vi "XYZStage-Read speed setting command.vi"(8 "error in (no error)":errorcluster, 9 "XYZ Stage data to queue":T2={"Command"=enum."Initialize", "Channel"="Z", "X"=0.0, "Y"=0.0, "Z"=0.0, "Speed"=0, "Zero"=FALSE, "Use acknowledgement?"=TRUE} {"Speed" format="Speed= %.0f"; "Z" format="Z= %#_g"; "Y" format="Y= %#_g"; "X" format="X= %#_g"}, 10 "Z Stage":T1, 11 "XY Stage config cluster":T5) -> (0 "error out":errorcluster)   [LabVIEW 2020]
doc: "Reads the XYZ Stage coordinates"
uses:
  Typedefs/XY Stage config cluster.ctl
  Typedefs/XYZ stage data.ctl
  Typedefs/XYZ stage states.ctl
  Typedefs/XYZ channel ring.ctl
  Typedefs/Z Stage config cluster.ctl
  Typedefs/Command acknowledgment states.ctl
  Global Variables/General Globals.vi
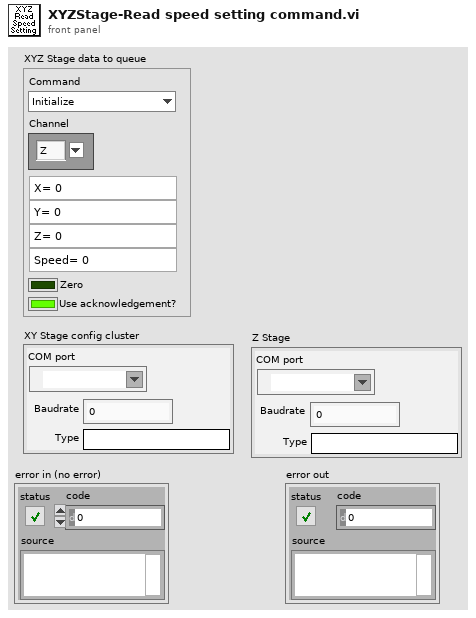
[diagram p1: front panel]
types:
  T1 = typedef "Z Stage config cluster.ctl" = cluster{"COM port":refnum<visa-resource-name>, "Baudrate":i32, "Type":string}
  T2 = typedef "XYZ stage data.ctl" = cluster{"Command":T3, "Channel":T4, "X":sgl, "Y":sgl, "Z":sgl, "Speed":i32, "Zero":bool, "Use acknowledgement?":bool}
  T3 = typedef "XYZ stage states.ctl" = enum16{"Dequeue", "Initialize", "Read Position", "Read Speed Setting", "Move", "Set Max Speed", "Reset Axis", "Stop all movement"}
  T4 = typedef "XYZ channel ring.ctl" = string
  T5 = typedef "XY Stage config cluster.ctl" = cluster{"COM port":refnum<visa-resource-name>, "Baudrate":i32, "Type":string}
  T6 = typedef "Command acknowledgment states.ctl" = enum16{"Acknowledge", "Wait for acknowledgment", "Release queue"}
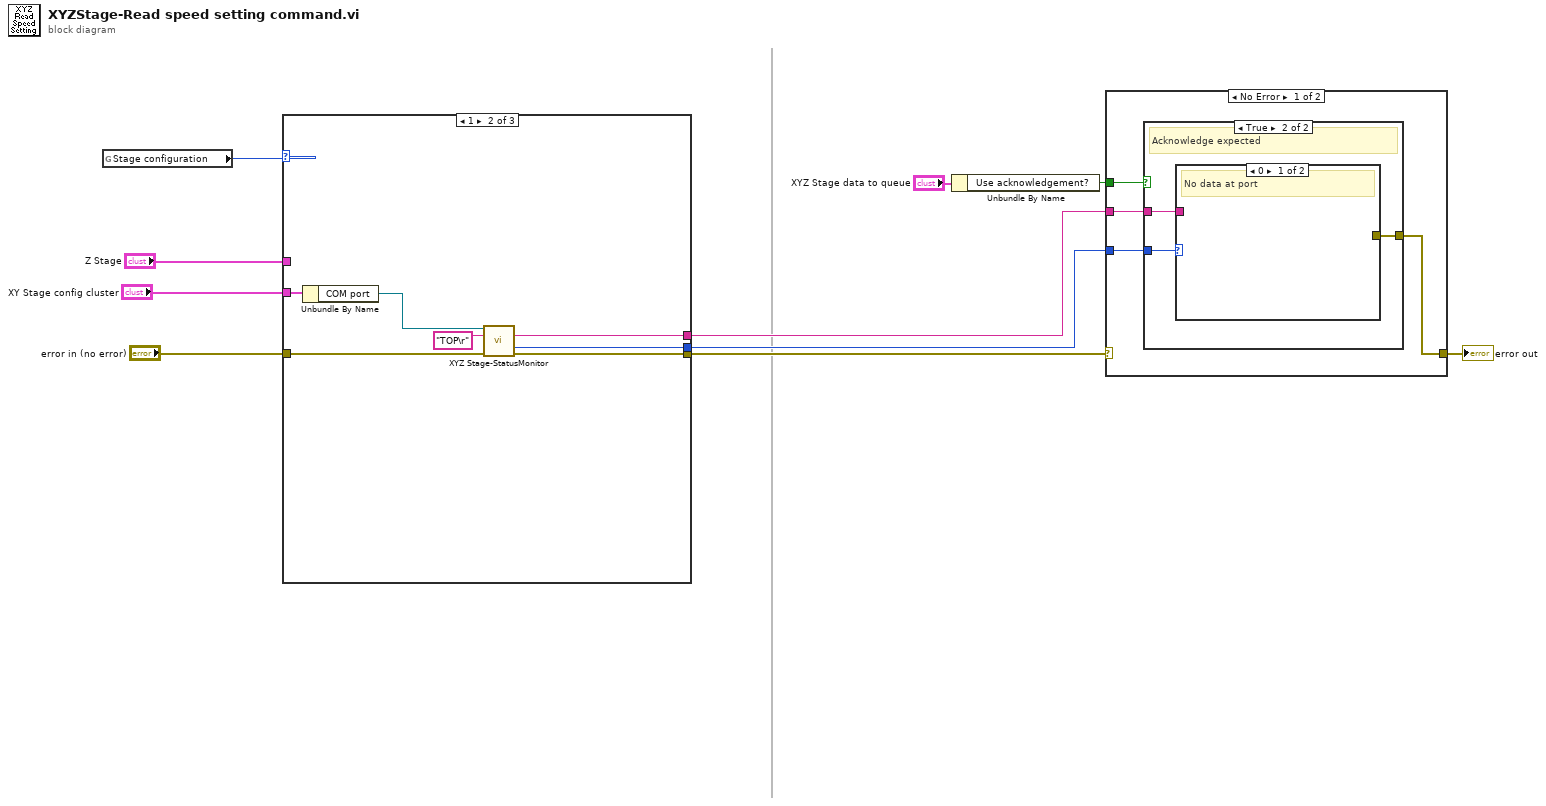
[diagram p0: block diagram]
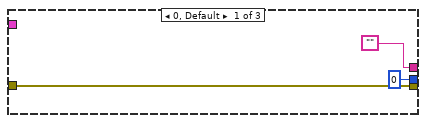
[diagram p2: hidden frame]
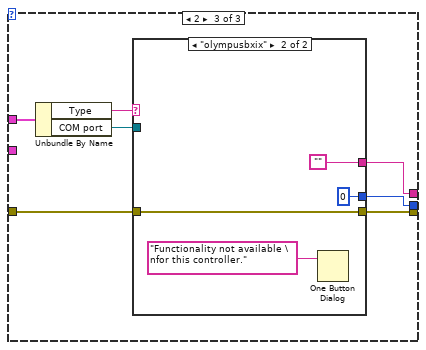
[diagram p3: hidden frame]
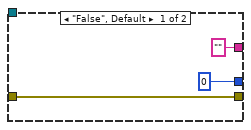
[diagram p4: hidden frame]
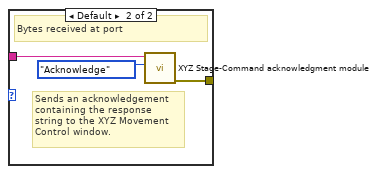
[diagram p6: hidden frame]
diagram:
  n1 = global read "General Globals.vi" "Stage configuration"() -> (w3:i32)
  n2 = case shown="1" w3 {
    tunnel: "error in (no error)" -> [w13 w20 w27]
    tunnel: ["" w18 w21] -> w7
    tunnel: [w13 w17 w26] -> w6
    tunnel: [u32 0 ("bytes read") w16 w22] -> w4
    tunnel: "Z Stage" -> [_ _ w25]
    tunnel: "XY Stage config cluster" -> [_ w15 _]
    frame 0, Default {
    }
    frame 1 {
      n3 = Unbundle By Name(w15) -> ("COM port"=w14:refnum<visa-resource-name>)
      n4 = call "XYZ Stage-StatusMonitor.vi"("VISA resource name"=w14, "string to write"="TOP\r", "Error In"=w20) -> ("read string"=w18:string, "bytes read"=w16:u32, "Error Out"=w17:errorcluster)  [unwired: 8 in, 2 out]
    }
    frame 2 {
      n5 = Unbundle By Name(w25) -> ("Type"=w23:string, "COM port"=w24:refnum<visa-resource-name>)
      n6 = case shown="\"olympusbxix\"" w23 {
        tunnel: w27 -> [w30 w34]
        tunnel: [w30 w34] -> w26
        tunnel: w24 -> [_ _]
        tunnel: [0 0] -> w22
        tunnel: ["" ""] -> w21
        frame "False", Default {
        }
        frame "olympusbxix" {
          n7 = One Button Dialog(message="Functionality not available \nfor this controller.") -> ()  [unwired: 1 in, 1 out]
        }
      }
    }
  }
  n8 = Unbundle By Name("XYZ Stage data to queue") -> ("Use acknowledgement?"=w9:bool)
  n9 = case shown="No Error" w6 {
    selector: w6 -> [_ w45]
    tunnel: w9 -> [w38 _]
    tunnel: w7 -> [w37 _]
    tunnel: [w36 w45] -> w5
    tunnel: w4 -> [w35 _]
    frame No Error {
      n10 = case shown="True" w38 {
        tunnel: w37 -> [_ w41]
        tunnel: [_ w40] -> w36
        tunnel: w35 -> [_ w39]
        frame False {
          # "No acknowledgement expected"
        }
        frame True {
          # "Acknowledge expected"
          n11 = case shown="0" w39 {
            tunnel: w41 -> [_ w43]
            tunnel: [_ w42] -> w40
            frame 0 {
              # "No data at port"
            }
            frame Default {
              # "Sends an acknowledgement containing the response string to the XYZ Movement Control window."
              # "Bytes received at port"
              n12 = call "XYZ Stage-Command acknowledgment module.vi"("State"=Command_acknowledgment_states."Acknowledge", "Acknowledgement Message in"=w43) -> ("error out"=w42:errorcluster)  [unwired: 7 in, 2 out]
            }
          }
        }
      }
    }
    frame Error {
    }
  }
  "error out" <- w5
